vi "Add Calculate Channel_Average_Average.vi"(7 "SysDef Ref":T1, 8 "error in (error out)":errorcluster, 9 "Average Settings":T2={"Name"="", "Description"="", "NumberOfPoints"=10, "Channel Node Path"="", "Alias Name"=""}, 11 "Calculated Channels Ref":refnum<k24>) -> (0 "error out":errorcluster, 3 "Calculated Channels Ref Out":refnum<k24>)   [LabVIEW 2019, in "Simple SysDef API.lvlib"]
uses:
  <userlib>/SimpleSysDef/Simple SysDef API.lvlib
  NationalInstruments.VeriStand.SystemDefinitionAPI
  <userlib>/SimpleSysDef/_SubVIs/Add Calculate Channel_Average_Settings.ctl
  <userlib>/SimpleSysDef/_SubVIs/System Definition Reference.ctl
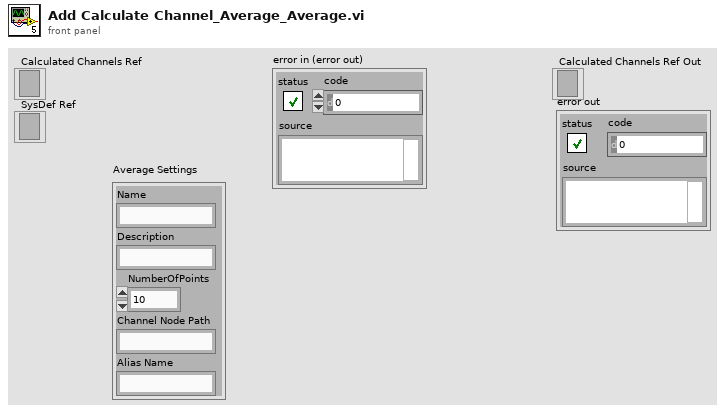
[diagram p1: front panel]
types:
  T1 = typedef "Simple SysDef API.lvlib/System Definition Reference.ctl" = refnum<k24>
  T2 = typedef "Simple SysDef API.lvlib/Add Calculate Channel_Average_Settings.ctl" = cluster{"Name":string, "Description":string, "NumberOfPoints":u32, "Channel Node Path":string, "Alias Name":string}
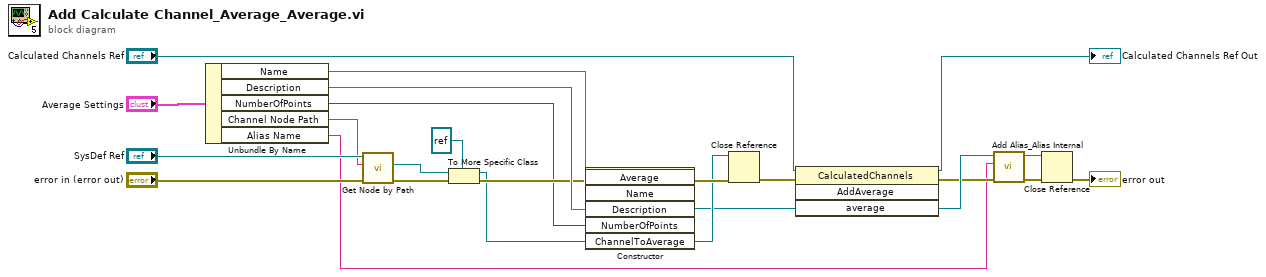
[diagram p0: block diagram]
diagram:
  n1 = Unbundle By Name("Average Settings") -> ("Name"=w14:string, "Description"=w13:string, "NumberOfPoints"=w7:u32, "Channel Node Path"=w8:string, "Alias Name"=w1:string)
  n2 = call <userlib>:"Get Node by Path.vi"("error in (no error)"="error in (error out)", "System Definition Node Path"=w8, "SysDef Ref"="SysDef Ref") -> ("error out"=w10:errorcluster, "Node Ref"=w11:refnum<k24>)  [unwired: 6 in, 1 out]
  n3 = To More Specific Class(target class=refnum<k24> refnum ("ChannelToAverage"), reference=w11, error in=w10) -> (specific class reference=w6:refnum<k24>, error out=w9:errorcluster)
  n4 = constructor class="Average"(error in=w9, "Name"=w14, "Description"=w13, "NumberOfPoints"=w7, "ChannelToAverage"=w6) -> (reference out=w5:refnum<k24>, error out=w16:errorcluster)  [unwired: 2 in, 5 out]
  n5 = Close Reference(reference=w6, error in (no error)=w16) -> (error out=w15:errorcluster)
  n6 = invoke class="CalculatedChannels" method="AddAverage"(reference="Calculated Channels Ref", error in=w15, "average"=w5) -> (reference out=→"Calculated Channels Ref Out":refnum<k24>, error out=w3:errorcluster)  [unwired: 1 in, 2 out]
  n7 = call <userlib>:"Add Alias_Alias Internal.vi"("error in (no error)"=w3, "Name"=w1, "Base Node"=w5) -> ("error out"=w2:errorcluster, "Base Node out"=w4:refnum<k24>)  [unwired: 7 in]
  n8 = Close Reference(reference=w4, error in (no error)=w2) -> (error out=→"error out":errorcluster)
